vi "max_min.vi"() -> ()   [LabVIEW 2019]
panel:
  in  "y":dbl
  in  "x":dbl
  out "min(x,y)":dbl
  out "max(x,y)":dbl
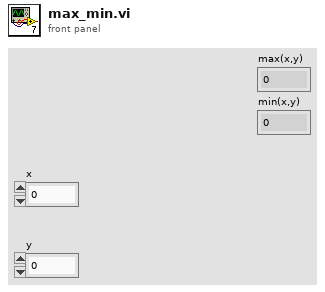
[diagram p1: front panel]
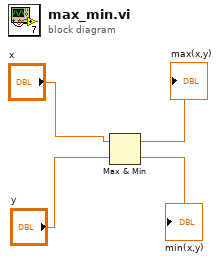
[diagram p0: block diagram]
diagram:
  n1 = Max & Min(x="x", y="y") -> (max(x,y)=→"max(x,y)":dbl, min(x,y)=→"min(x,y)":dbl)
